vi "ASyncIO.vi"() -> ()   [LabVIEW 2018]
uses:
  <vilib>/Instr/_visa.llb/VISA Configure Serial Port (Instr).vi
  <vilib>/LabVIEW Interface for Arduino/LabVIEW Interface for Arduino.lvlib
panel:
  out "Waveform Chart":dynamicdata(graph)
  out "Voltage":dbl(slide) scale=0.0..5.0
  out "Blue On?":bool
  out "Green On?":bool
  in  "Blue LED":bool
  in  "Green LED":bool
  out "Arduino COM port":refnum<visa-resource-name>
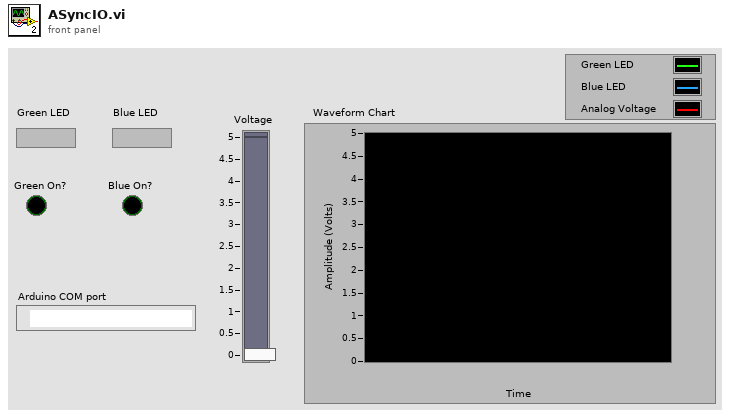
[diagram p1: front panel]
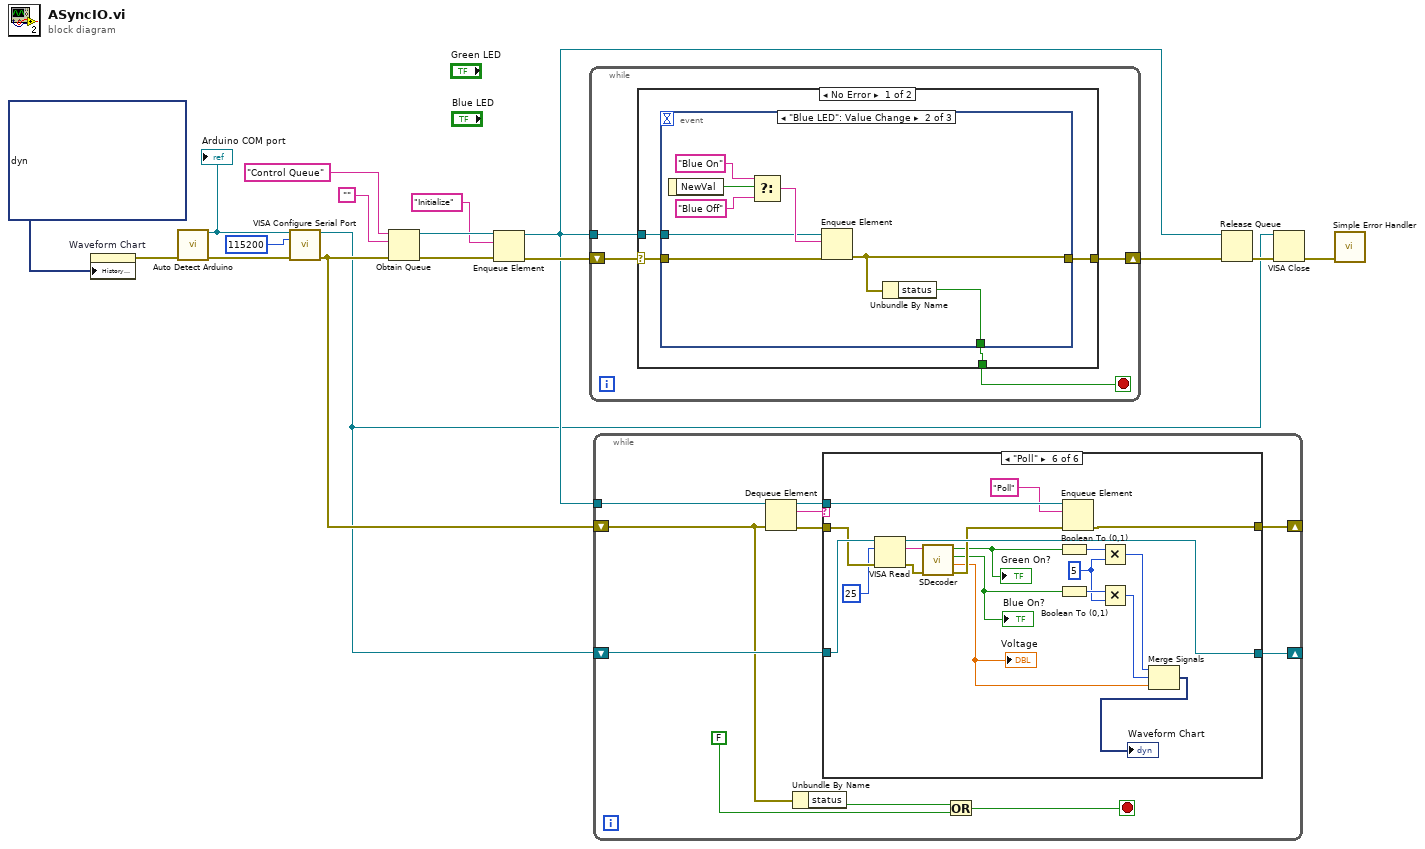
[diagram p0: block diagram]
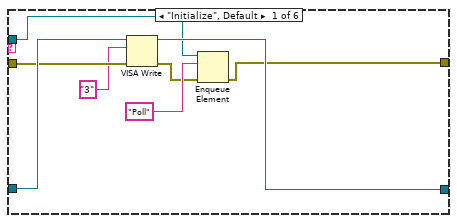
[diagram p2: hidden frame]
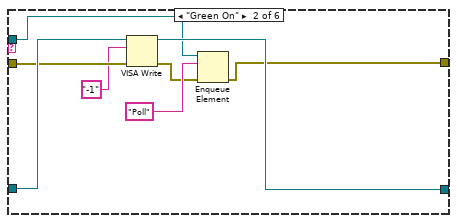
[diagram p3: hidden frame]
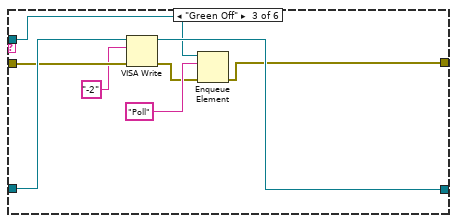
[diagram p4: hidden frame]
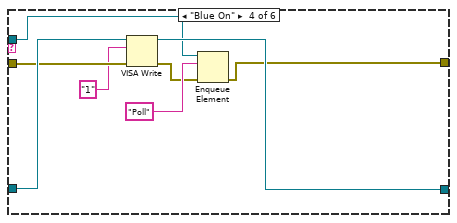
[diagram p5: hidden frame]
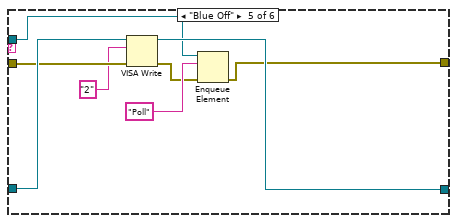
[diagram p6: hidden frame]
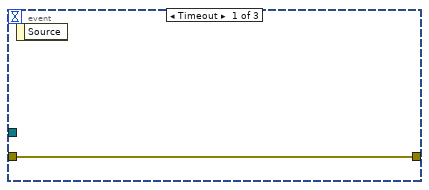
[diagram p7: hidden frame]
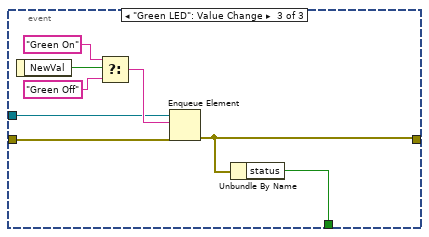
[diagram p8: hidden frame]
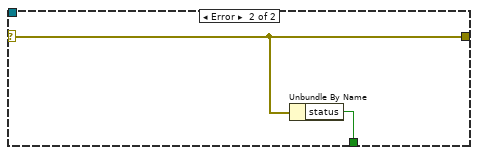
[diagram p9: hidden frame]
diagram:
  n1 = property on="Waveform Chart" class="WFChart (strict)"("History Data"=dynamicdata[] [[{"t0"=timestamp(34618050000 s since 1904-01-01), "dt"=1.0, "Y"=[]}]]) -> (error out=w2:errorcluster)  [unwired: 2 in, 1 out]
  n2 = call <vilib>:"Auto Detect Arduino.vi"("error in (no error)"=w2) -> ("VISA resource"=w11:refnum<visa-resource-name>, "error out"=w10:errorcluster)  [unwired: 13 in]
  "Arduino COM port" <- w11
  n3 = call-poly "VISA Configure Serial Port"("VISA resource name"=w11, "baud rate (9600)"=115200, "error in (no error)"=w10) -> ("VISA resource name out"=w4:refnum<visa-resource-name>, "error out"=w8:errorcluster)  [unwired: 11 in]
  n4 = Obtain Queue(name (unnamed)="Control Queue", element data type="", error in (no error)=w8) -> (queue out=w15:refnum<queue>, error out=w14:errorcluster)  [unwired: 2 in, 1 out]
  n5 = Enqueue Element(queue=w15, element="Initialize", error in (no error)=w14) -> (queue out=w6:refnum<queue>, error out=w13:errorcluster)  [unwired: 1 in, 1 out]
  n6 = while {
    tunnel: w6 -> [w18]
    shift-right: [w20] -> w12
    shift-left: w13 -> [w21]
    stop <- w19 stop-if-true
    n7 = case shown="No Error" w21 {
      selector: w21 -> [w25 w44]
      tunnel: [w24 w44] -> w20
      tunnel: [w22 w43] -> w19
      tunnel: w18 -> [w23 _]
      frame No Error {
        n8 = event shown="[1] \"Blue LED\": Value Change" {
          selector: _ -> [_ _ _]
          dyn-events: _ -> [_ _ _]
          timeout: _ -> [_ _ _]
          tunnel: w25 -> [w26 w29 w37]
          tunnel: [w26 w28 w36] -> w24
          tunnel: w23 -> [_ w30 w38]
          tunnel: [_ w27 w35] -> w22
          event Timeout {
            n9 = event-data() -> ()  [unwired: 1 in, 1 out]
          }
          event "Blue LED": Value Change {
            n10 = event-data() -> ("NewVal"=w34:bool)  [unwired: 1 in]
            n11 = Select(t="Blue On", s=w34, f="Blue Off") -> (s? t:f=w31:string)
            n12 = Enqueue Element(queue=w30, element=w31, error in (no error)=w29) -> (error out=w28:errorcluster)  [unwired: 1 in, 2 out]
            n13 = Unbundle By Name(w28) -> ("status"=w27:bool)
          }
          event "Green LED": Value Change {
            n14 = event-data() -> ("NewVal"=w42:bool)  [unwired: 1 in]
            n15 = Select(t="Green On", s=w42, f="Green Off") -> (s? t:f=w39:string)
            n16 = Enqueue Element(queue=w38, element=w39, error in (no error)=w37) -> (error out=w36:errorcluster)  [unwired: 1 in, 2 out]
            n17 = Unbundle By Name(w36) -> ("status"=w35:bool)
          }
        }
      }
      frame Error {
        n18 = Unbundle By Name(w44) -> ("status"=w43:bool)
      }
    }
  }
  n19 = while {
    tunnel: w6 -> [w45]
    shift-right: [w52] -> _
    shift-left: w8 -> [w46]
    shift-right: [w51] -> _
    shift-left: w4 -> [w54]
    stop <- w47 stop-if-true
    n20 = Dequeue Element(queue=w45, error in (no error)=w46) -> (queue out=w50:refnum<queue>, element=w55:string, error out=w53:errorcluster)  [unwired: 1 in, 1 out]
    n21 = Unbundle By Name(w46) -> ("status"=w49:bool)
    n22 = case shown="\"Poll\"" w55 {
      tunnel: w54 -> [w63 w71 w79 w87 w95 w111]
      tunnel: w53 -> [w62 w70 w78 w86 w94 w110]
      tunnel: [w57 w65 w73 w81 w89 w113] -> w52
      tunnel: [w60 w68 w76 w84 w92 w109] -> w51
      tunnel: w50 -> [w59 w67 w75 w83 w91 w114]
      frame "Initialize", Default {
        n23 = VISA Write(VISA resource name=w63, write buffer="3", error in (no error)=w62) -> (VISA resource name out=w60:refnum<visa-resource-name>, error out=w56:errorcluster)  [unwired: 1 out]
        n24 = Enqueue Element(queue=w59, element="Poll", error in (no error)=w56) -> (error out=w57:errorcluster)  [unwired: 1 in, 2 out]
      }
      frame "Green On" {
        n25 = VISA Write(VISA resource name=w71, write buffer="-1", error in (no error)=w70) -> (VISA resource name out=w68:refnum<visa-resource-name>, error out=w64:errorcluster)  [unwired: 1 out]
        n26 = Enqueue Element(queue=w67, element="Poll", error in (no error)=w64) -> (error out=w65:errorcluster)  [unwired: 1 in, 2 out]
      }
      frame "Green Off" {
        n27 = VISA Write(VISA resource name=w79, write buffer="-2", error in (no error)=w78) -> (VISA resource name out=w76:refnum<visa-resource-name>, error out=w72:errorcluster)  [unwired: 1 out]
        n28 = Enqueue Element(queue=w75, element="Poll", error in (no error)=w72) -> (error out=w73:errorcluster)  [unwired: 1 in, 2 out]
      }
      frame "Blue On" {
        n29 = VISA Write(VISA resource name=w87, write buffer="1", error in (no error)=w86) -> (VISA resource name out=w84:refnum<visa-resource-name>, error out=w80:errorcluster)  [unwired: 1 out]
        n30 = Enqueue Element(queue=w83, element="Poll", error in (no error)=w80) -> (error out=w81:errorcluster)  [unwired: 1 in, 2 out]
      }
      frame "Blue Off" {
        n31 = VISA Write(VISA resource name=w95, write buffer="2", error in (no error)=w94) -> (VISA resource name out=w92:refnum<visa-resource-name>, error out=w88:errorcluster)  [unwired: 1 out]
        n32 = Enqueue Element(queue=w91, element="Poll", error in (no error)=w88) -> (error out=w89:errorcluster)  [unwired: 1 in, 2 out]
      }
      frame "Poll" {
        w100 = 5
        n33 = VISA Read(VISA resource name=w111, byte count=25, error in (no error)=w110) -> (VISA resource name out=w109:refnum<visa-resource-name>, read buffer=w108:string, error out=w107:errorcluster)  [unwired: 1 out]
        n34 = call "SDecoder.vi"("error in (no error)"=w107, "Input String"=w108) -> ("error out"=w106:errorcluster, "Measured Volts"=w97:dbl, "Blue On?"=w102:bool, "Green On?"=w103:bool)  [unwired: 6 in]
        "Green On?" <- w103
        "Blue On?" <- w102
        "Voltage" <- w97
        n35 = Boolean To (0,1)(Boolean=w103) -> (0, 1=w104:i16)
        n36 = Boolean To (0,1)(Boolean=w102) -> (0, 1=w101:i16)
        n37 = Enqueue Element(queue=w114, element="Poll", error in (no error)=w106) -> (error out=w113:errorcluster)  [unwired: 1 in, 2 out]
        n38 = Multiply(x=w104, y=w100) -> (x*y=w99:i32)
        n39 = Multiply(x=w101, y=w100) -> (x*y=w98:i32)
        n40 = Merge Signals(w99, w98, w97) -> (→"Waveform Chart":dynamicdata)
      }
    }
    n41 = Or(x=w49, y=FALSE) -> (x .or. y?=w47:bool)
  }
  n42 = Release Queue(queue=w6, error in (no error)=w12) -> (error out=w5:errorcluster)  [unwired: 1 in, 2 out]
  n43 = VISA Close(VISA resource name=w4, error in (no error)=w5) -> (error out=w3:errorcluster)
  n44 = call <vilib>:"Simple Error Handler.vi"("error in (no error)"=w3) -> ()  [unwired: 4 in, 5 out]
